vi "Hold Jobber in Memory.vi"() -> ()   [LabVIEW 2014]
uses:
  Classes/Job/Job.lvclass
  Actors/Jobber/Jobber/Jobber.lvclass
  <vilib>/ActorFramework/Actor/Actor.lvclass
  <vilib>/ActorFramework/Message Enqueuer/Message Enqueuer.lvclass
  <vilib>/ActorFramework/Message/Message.lvclass
  <vilib>/ActorFramework/Lower Proxy Actor/Lower Proxy Actor.lvclass
  <vilib>/ActorFramework/Proxy Actor/Proxy Actor.lvclass
panel:
  in  "Boolean":bool
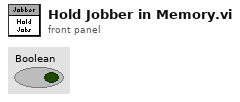
[diagram p1: front panel]
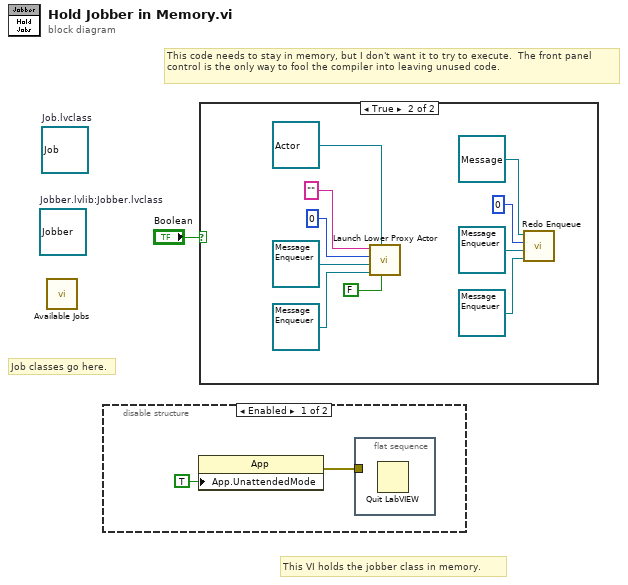
[diagram p0: block diagram]
diagram:
  (unwired) refnum<class "Jobber.lvclass"> refnum  # Jobber.lvlib:Jobber.lvclass
  (unwired) refnum<class "Job.lvclass"> refnum  # Job.lvclass
  # "Job classes go here."
  # "This code needs to stay in memory, but I don't want it to try to execute.  The front panel control is the only way to fool the compiler into leaving unused code."
  # "This VI holds the jobber class in memory."
  n1 = call "Available Jobs.vi"() -> ()  [unwired: 12 in]
  n2 = disable-structure shown="Enabled" {
    frame Enabled {
      n3 = property class="App"("App.UnattendedMode"=TRUE ("Application:Unattended Mode")) -> (error out=w2:errorcluster)  [unwired: 2 in, 1 out]
      n4 = flat-sequence {
        tunnel: w2 -> [_]
        frame #0 {
          n5 = Quit LabVIEW() -> ()  [unwired: 1 in]
        }
      }
    }
    frame Disabled {
    }
  }
  n6 = case shown="True" "Boolean" {
    frame False {
    }
    frame True {
      n7 = call <vilib>:"Launch Lower Proxy Actor.vi"("Open Actor Core front panel? (F)"=FALSE, "Real Actor"=refnum<class "Actor.lvclass"> refnum, "Upper Proxy Enqueuer"=refnum<class "Message Enqueuer.lvclass"> refnum, "Caller Enqueuer"=refnum<class "Message Enqueuer.lvclass"> refnum, "Server Port"=u32 0, "Machine IP"="") -> ()  [unwired: 4 in, 2 out]
      n8 = call <vilib>:"Redo Enqueue.vi"("Opposite Proxy Enqueuer"=refnum<class "Message Enqueuer.lvclass"> refnum, "Real Enqueuer"=refnum<class "Message Enqueuer.lvclass"> refnum, "priority"=0, "Message"=refnum<class "Message.lvclass"> refnum) -> ()  [unwired: 7 in, 1 out]
    }
  }
